vi "Enemy_Robot.vi"(8 "error in":errorcluster, 9 "Array":u8[](array[numeric]) format="%02x") -> (0 "error out":errorcluster, 1 "array w/ subset deleted":u8[](array[numeric]), 3 "Enemy_Robots":T1)   [LabVIEW 2017]
uses:
  Varint Decoder uint32.vi
panel:
  in  "Enemy_robots":T1
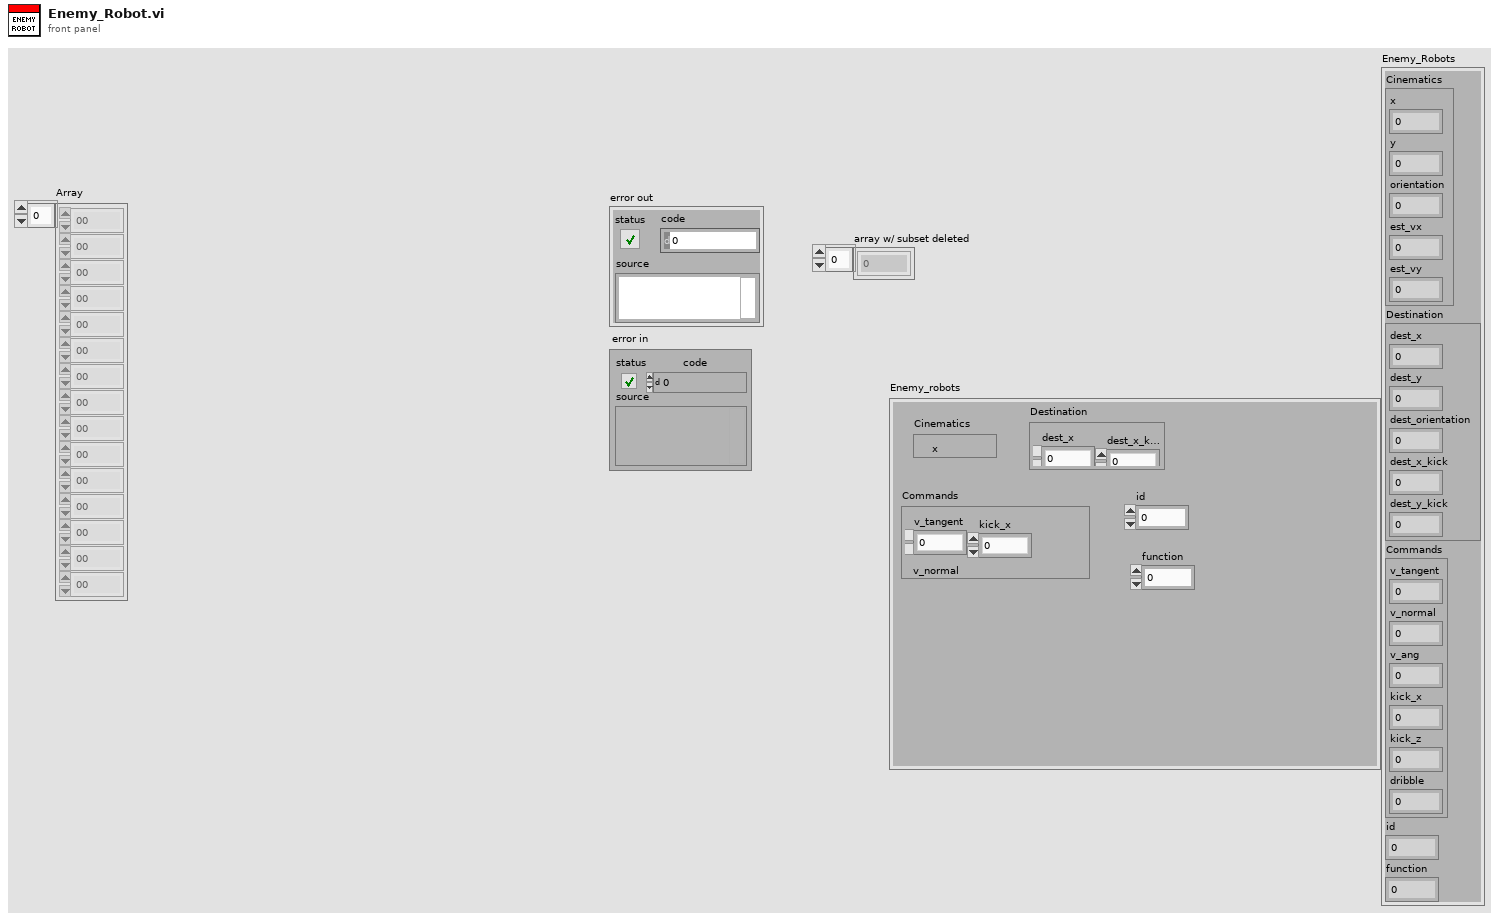
[diagram p1: front panel]
types:
  T1 = cluster{"Cinematics":cluster{"x":dbl, "y":dbl, "orientation":dbl, "est_vx":dbl, "est_vy":dbl}, "Destination":cluster{"dest_x":dbl, "dest_y":dbl, "dest_orientation":dbl, "dest_x_kick":dbl, "dest_y_kick":dbl}, "Commands":cluster{"v_tangent":dbl, "v_normal":dbl, "v_ang":dbl, "kick_x":dbl, "kick_z":dbl, "dribble":u32}, "id":u32, "function":u32}
  T2 = cluster{"x":dbl, "y":dbl, "orientation":dbl, "est_vx":dbl, "est_vy":dbl}
  T3 = cluster{"dest_x":dbl, "dest_y":dbl, "dest_orientation":dbl, "dest_x_kick":dbl, "dest_y_kick":dbl}
  T4 = cluster{"v_tangent":dbl, "v_normal":dbl, "v_ang":dbl, "kick_x":dbl, "kick_z":dbl, "dribble":u32}
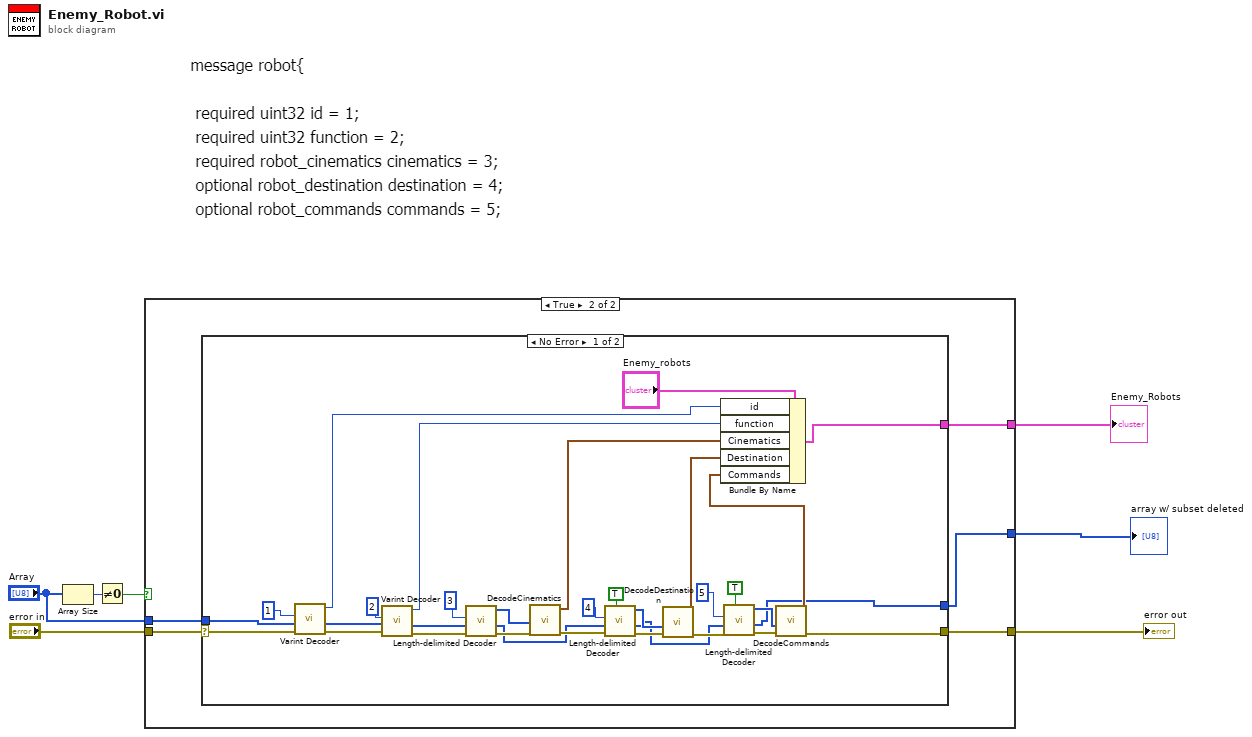
[diagram p0: block diagram]
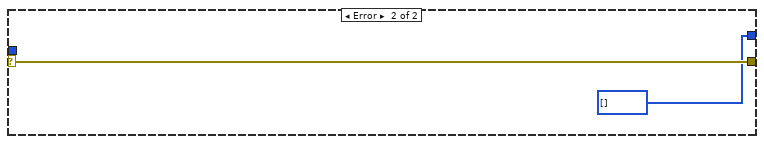
[diagram p3: hidden frame]
diagram:
  n1 = Array Size(array="Array") -> (size(s)=w5:i32)
  n2 = Not Equal To 0?(x=w5) -> (x != 0?=w3:bool)
  n3 = case shown="True" w3 {
    tunnel: "error in" -> [_ w12]
    tunnel: "Array" -> [_ w11]
    tunnel: [_ w10] -> w4
    tunnel: [_ w9] -> w2
    tunnel: [_ w8] -> w1
    frame False {
    }
    frame True {
      n4 = case shown="No Error" w12 {
        selector: w12 -> [w43 w46]
        tunnel: [w26 w46] -> w10
        tunnel: [w13 u8[] [] ("array w/ subset deleted")] -> w9
        tunnel: w11 -> [w42 _]
        tunnel: [w19 _] -> w8
        frame No Error {
          n5 = call-poly "Varint Decoder.vi"("error in (no error)"=w43, "Array"=w42, "Key"=1) -> ("error out"=w41:errorcluster, "array w/ subset deleted"=w40:u8[], "Varint"=w24:u32)  [unwired: 5 in, 1 out]
          n6 = call-poly "Varint Decoder.vi"("error in (no error)"=w41, "Array"=w40, "Key"=2) -> ("error out"=w37:errorcluster, "array w/ subset deleted"=w38:u8[], "Varint"=w23:u32)  [unwired: 5 in, 1 out]
          n7 = call "Length-delimited Decoder.vi"("error in (no error)"=w37, "Array"=w38, "Key"=3) -> ("error out"=w35:errorcluster, "array w/ subset deleted"=w17:u8[], "Length-delimited"=w18:u8[])  [unwired: 5 in, 1 out]
          n8 = call "DecodeCinematics.vi"("error in"=w35, "Array"=w18) -> ("error out"=w34:errorcluster, "Cinematics"=w22:T2)  [unwired: 7 in, 1 out]
          n9 = call "Length-delimited Decoder.vi"("Optional"=TRUE, "error in (no error)"=w34, "Array"=w17, "Key"=4) -> ("error out"=w31:errorcluster, "array w/ subset deleted"=w15:u8[], "Length-delimited"=w16:u8[])  [unwired: 4 in, 1 out]
          n10 = call "DecodeDestination.vi"("error in"=w31, "Array"=w16) -> ("error out"=w30:errorcluster, "Destination"=w21:T3)  [unwired: 7 in, 1 out]
          n11 = call "Length-delimited Decoder.vi"("Optional"=TRUE, "error in (no error)"=w30, "Array"=w15, "Key"=5) -> ("error out"=w27:errorcluster, "array w/ subset deleted"=w13:u8[], "Length-delimited"=w14:u8[])  [unwired: 4 in, 1 out]
          n12 = call "DecodeCommands.vi"("error in"=w27, "Array"=w14) -> ("error out"=w26:errorcluster, "Commands"=w20:T4)  [unwired: 7 in, 1 out]
          n13 = Bundle By Name(cluster="Enemy_robots", "id"=w24, "function"=w23, "Cinematics"=w22, "Destination"=w21, "Commands"=w20) -> (w19:T1)
        }
        frame Error {
        }
      }
    }
  }
  "error out" <- w4
  "array w/ subset deleted" <- w2
  "Enemy_Robots" <- w1
